vi "ErrorHandler.vi"(8 "error in":errorcluster, 9 "Custom Message":string, 11 "AIM Error":i32) -> (0 "error out":errorcluster)   [LabVIEW 2020, in "AIM664LV.lvlib"]
uses:
  AIM664LV.lvlib
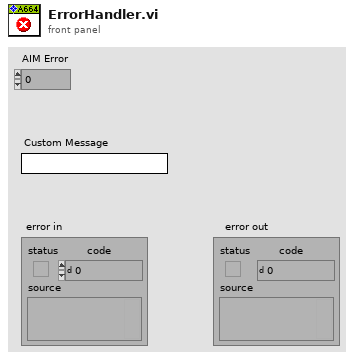
[diagram p1: front panel]
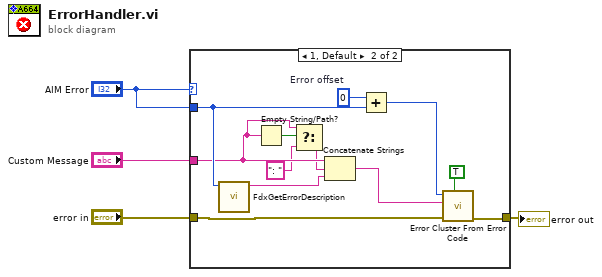
[diagram p0: block diagram]
diagram:
  n1 = case shown="1, Default" "AIM Error" {
    tunnel: "error in" -> [w5 w17]
    tunnel: [w5 w16] -> w3
    tunnel: "Custom Message" -> [_ w8]
    tunnel: "AIM Error" -> [_ w14]
    frame 0 {
    }
    frame 1, Default {
      w13 = 0  # Error offset
      n2 = call "FdxGetErrorDescription.vi"("fdx_error_code"=w14) -> ("string description"=w11:string)  [unwired: 9 in, 1 out]
      n3 = Empty String/Path?(string/path=w8) -> (empty?=w9:bool)
      n4 = Select(t=w8, s=w9, f=": " ("string")) -> (s? t:f=w6:string)
      n5 = Concatenate Strings(w8, w6, w11) -> (w10:string)
      n6 = Add(x=w13, y=w14) -> (x+y=w12:i32)
      n7 = call <vilib>:"Error Cluster From Error Code.vi"("show call chain? (False)"=TRUE, "error in (no error)"=w17, "error message (\"\")"=w10, "error code (0)"=w12) -> ("error out"=w16:errorcluster)  [unwired: 5 in]
    }
  }
  "error out" <- w3
